vi "Move a Motor.vi"(7 "target pos mode":enum16{"backend", "frontend"}(ring), 8 "error in (no error)":errorcluster, 9 "target pos":dbl, 10 "Index":i32, 11 "Motions in":refnum<class "Motions.lvclass">) -> (0 "error out":errorcluster, 3 "Motions out":refnum<class "Motions.lvclass">)   [LabVIEW 2016, in "Hardware.lvlib" / "Motions.lvlib" / "Motions.lvclass"]
uses:
  <userlib>/Common Components/Hardware/Abstract System/Motions/Motions/Motions.lvclass
panel:
  # "target pos from FP may be different from the real pos, but with offset"
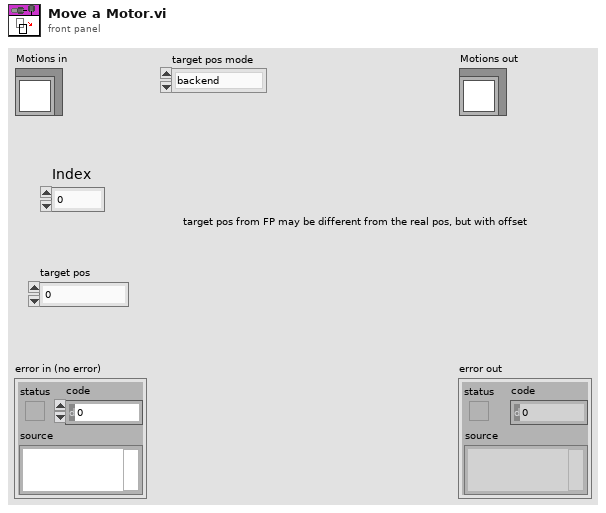
[diagram p1: front panel]
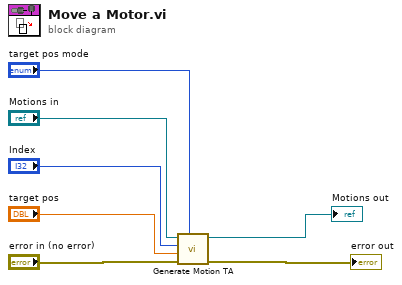
[diagram p0: block diagram]
diagram:
  n1 = call <userlib>:"Generate Motion TA.vi"("target pos mode"="target pos mode", "error in (no error)"="error in (no error)", "target pos"="target pos", "Index"="Index", "Motions in"="Motions in") -> ("error out"=→"error out":errorcluster, "Motions out"=→"Motions out":refnum<class "Motions.lvclass">)  [unwired: 5 in]
